vi "Test-1.vi"() -> ()   [LabVIEW 2020]
uses:
  Quick-GUI-Update/Quick-GUI-Update.lvclass
  fee3559f-63eb-40a2-ae3c-83a391cb0737.vi
panel:
  in  "Enum":enum16{"hai", "hello"}(ring)
  in  "string":string
  out "Status":u8[](array[numeric])
  out "Boolean":bool
  out "Label's List":string[][](array[string])
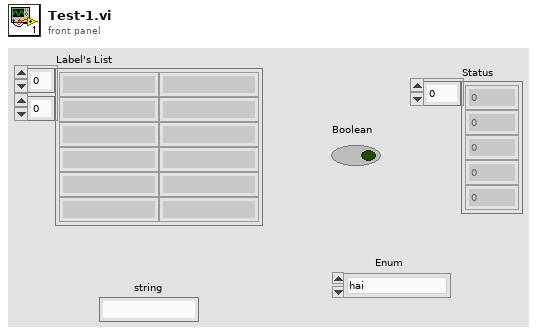
[diagram p1: front panel]
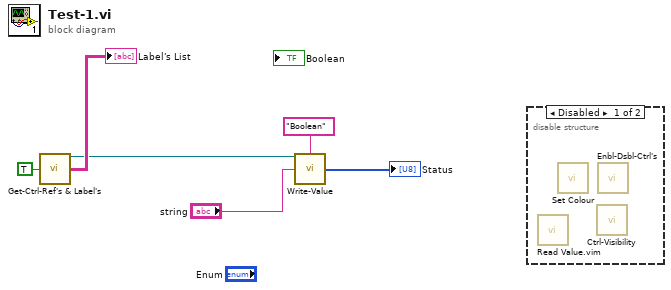
[diagram p0: block diagram]
diagram:
  n1 = call "Get-Ctrl-Ref's & Label's.vi"("Show All Label List"=TRUE) -> ("Quick-GUI-Update out"=w4:refnum<class "Quick-GUI-Update.lvclass">, "Label's List"=→"Label's List":string[][])  [unwired: 12 in, 1 out]
  n2 = call "Write-Value.vi"("Quick-GUI-Update in"=w4, "Label"="Boolean" ("Lable"), "Value In"="string") -> ("Status"=→"Status":u8[])  [unwired: 10 in, 2 out]
  n3 = disable-structure shown="Disabled" {
    frame Disabled {
      n4 = call "Read Value.vim"() -> ()  [unwired: 12 in, 4 out]
      n5 = call "Set Colour.vi"() -> ()  [unwired: 14 in, 2 out]
      n6 = call "Ctrl-Visibility.vi"() -> ()  [unwired: 14 in, 2 out]
      n7 = call "Enbl-Dsbl-Ctrl's.vi"() -> ()  [unwired: 14 in, 2 out]
    }
    frame Enabled {
    }
  }
